vi "Mecanum Drive.vi"(0 "X In":dbl, 5 "Y In":dbl, 7 "R In":dbl, 9 "Manual Override":bool, 11 "Reset Header":bool) -> (4 "X Out":dbl, 6 "Y Out":dbl, 8 "R Out":dbl)   [LabVIEW 2014]
uses:
  Global Variables/Refnum Names.vi
  <vilib>/addons/control/pid/pid.llb/PID (DBL).vi
  <vilib>/addons/control/pid/NI_PID_pid.lvlib
panel:
  out "Header":dbl
  out "Initialize Header":bool=TRUE
  in  "STRAIGHT PID":T1={"proportional gain (Kc)"=0.02, "integral time (Ti, min)"=0.05, "derivative time (Td, min)"=0.0} {"derivative time (Td, min)" format="%.3f"; "integral time (Ti, min)" format="%.3f"; "proportional gain (Kc)" format="%.3f"}
  out "PID Output":dbl format="%.2f"
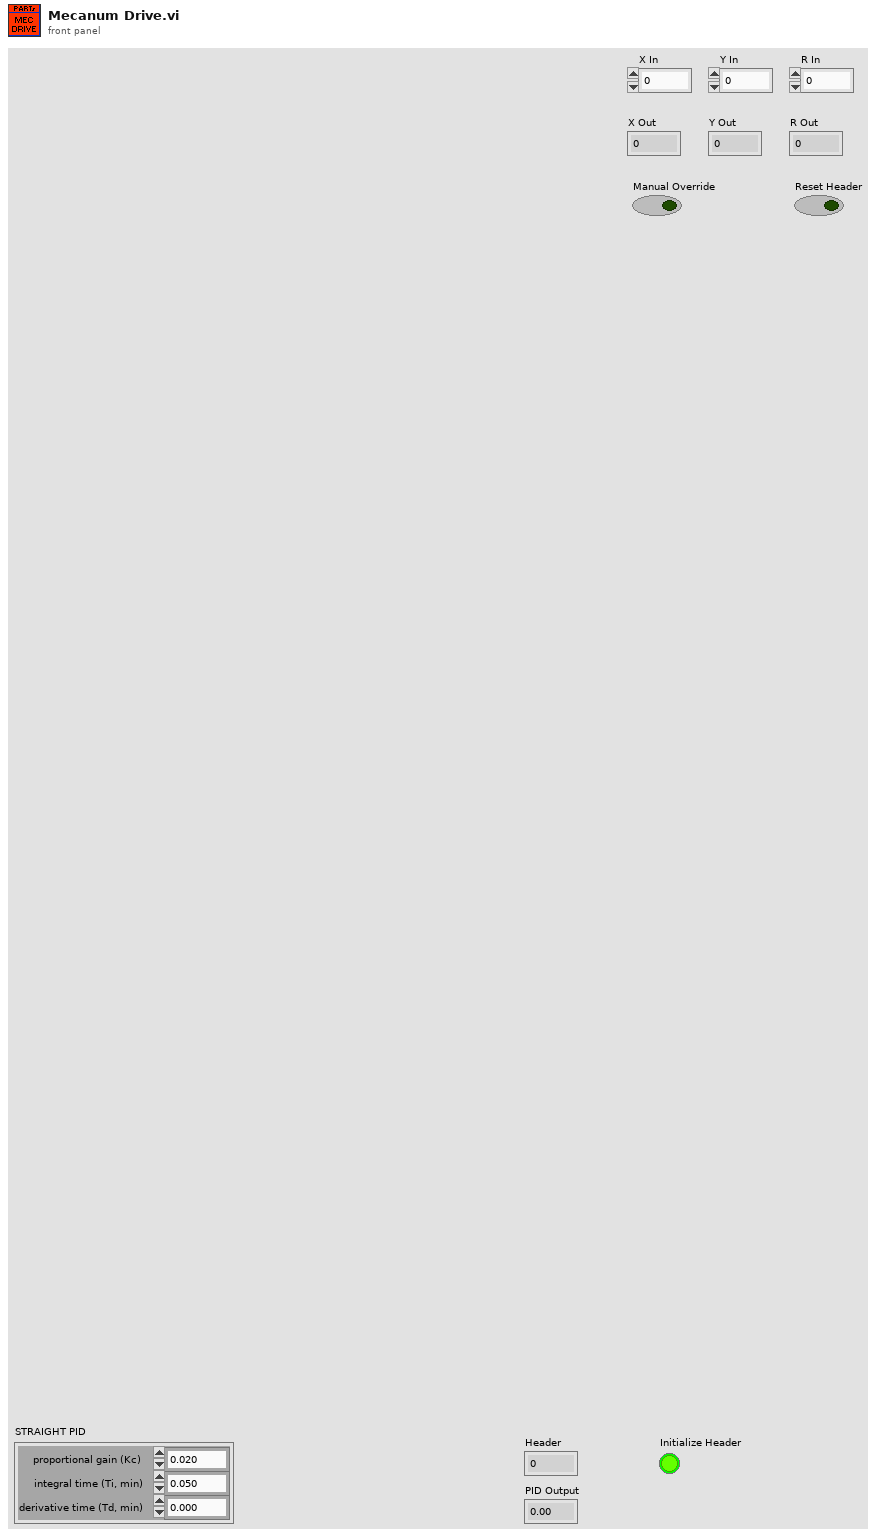
[diagram p1: front panel]
types:
  T1 = cluster{"proportional gain (Kc)":dbl, "integral time (Ti, min)":dbl, "derivative time (Td, min)":dbl}
  T2 = typedef "WPI_GyroDevRef.ctl" = cluster{"DevStatus":errorcluster, "Analog Module":T3, "Analog Channel":T4, "Offset":dbl, "Gain (VoltsPerDegree/Second)":dbl}
  T3 = typedef "FPGA_TypedefAnalogModule.ctl" = enum16{"Controller 1"}
  T4 = typedef "FPGA_AIChannel.ctl" = enum8{"AI 0", "AI 1", "AI 2", "AI 3", "AI MXP 0", "AI MXP 1", "AI MXP 2", "AI MXP 3", "Invalid"}
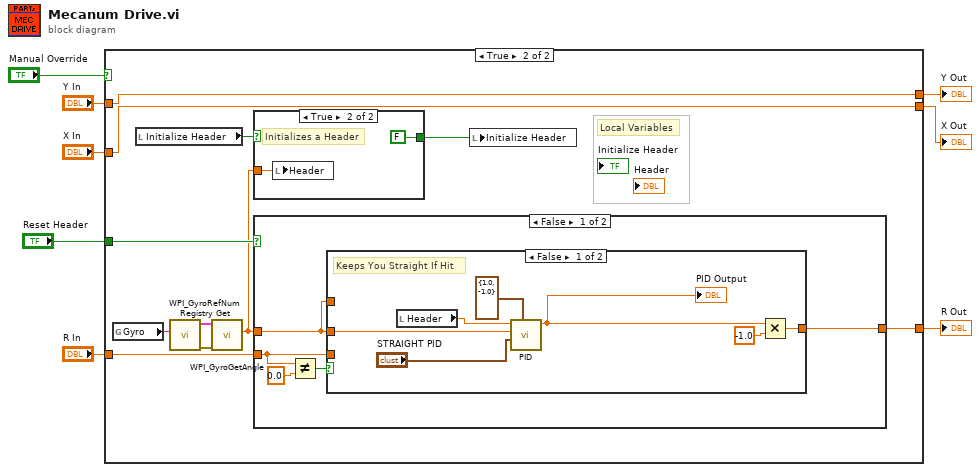
[diagram p0: block diagram]
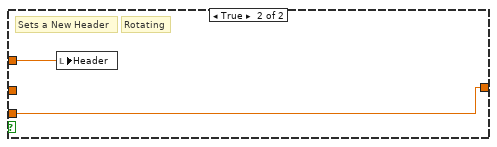
[diagram p3: hidden frame]
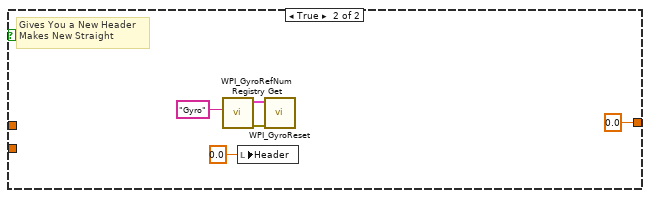
[diagram p4: hidden frame]
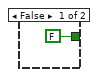
[diagram p5: hidden frame]
diagram:
  n1 = case shown="True" "Manual Override" {
    tunnel: [w9 w22] -> w2
    tunnel: "Y In" -> [w11 w13]
    tunnel: "X In" -> [w10 w14]
    tunnel: "Reset Header" -> [_ w19]
    tunnel: [w11 w13] -> w3
    tunnel: "R In" -> [w9 w15]
    tunnel: [w10 w14] -> w4
    frame False {
    }
    frame True {
      # "Local Variables"
      n2 = global read "Refnum Names.vi" "Gyro"() -> (w12:string)
      n3 = local read "Initialize Header"() -> (w21:bool)
      n4 = call <vilib>:"WPI_GyroRefNum Registry Get.vi"("refnum name"=w12) -> ("error out"=w16:errorcluster, "GyroDevRef"=w18:T2)  [unwired: 9 in]
      n5 = call <vilib>:"WPI_GyroGetAngle.vi"("error in (no error)"=w16, "GyroDevRef"=w18) -> ("Angle"=w17:dbl)  [unwired: 6 in, 3 out]
      n6 = case shown="True" w21 {
        tunnel: w17 -> [_ w44]
        tunnel: [FALSE FALSE] -> w20
        frame False {
        }
        frame True {
          # "Initializes a Header"
          n7 = local write "Header"(w44) -> ()
        }
      }
      n8 = case shown="False" w19 {
        tunnel: [w27 0.0] -> w22
        tunnel: w15 -> [w24 _]
        tunnel: w17 -> [w23 _]
        frame False {
          n9 = Not Equal?(x=w24, y=0.0) -> (x != y?=w25:bool)
          n10 = case shown="False" w25 {
            tunnel: [w33 w35] -> w27
            tunnel: w23 -> [w34 _]
            tunnel: w23 -> [_ w36]
            tunnel: w24 -> [_ w35]
            frame False {
              # "Keeps You Straight If Hit"
              n11 = local read "Header"() -> (w30:dbl)
              n12 = call-poly <vilib>:"PID.vi"("output range"=cluster{"output high":dbl, "output low":dbl} {"output high"=1.0, "output low"=-1.0}, "PID gains"="STRAIGHT PID", "process variable"=w34, "setpoint"=w30) -> ("output"=w29:dbl)  [unwired: 6 in, 1 out]
              "PID Output" <- w29
              n13 = Multiply(x=w29, y=-1.0) -> (x*y=w33:dbl)
            }
            frame True {
              # "Sets a New Header"
              # "Rotating"
              n14 = local write "Header"(w36) -> ()
            }
          }
        }
        frame True {
          # "Gives You a New Header\nMakes New Straight"
          n15 = call <vilib>:"WPI_GyroRefNum Registry Get.vi"("refnum name"="Gyro") -> ("error out"=w40:errorcluster, "GyroDevRef"=w39:T2)  [unwired: 9 in]
          n16 = local write "Header"(0.0 ("Header 2")) -> ()
          n17 = call <vilib>:"WPI_GyroReset.vi"("error in (no error)"=w40, "GyroDevRef"=w39) -> ()  [unwired: 8 in, 2 out]
        }
      }
      n18 = local write "Initialize Header"(w20) -> ()
    }
  }
  "X Out" <- w4
  "Y Out" <- w3
  "R Out" <- w2
